vi "S2C_CheckBuildScript.vi"(8 "Error In":errorcluster, 11 "Entry":string) -> (0 "Error Out":errorcluster, 3 "Data":string[](array[string]))   [LabVIEW 2015]
doc: "Converts a script line entry into an executable table entry."
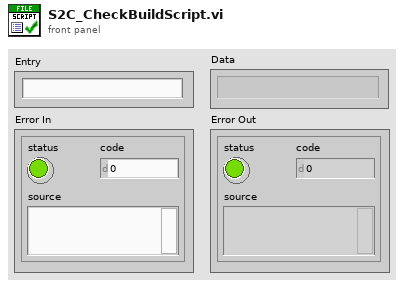
[diagram p1: front panel]
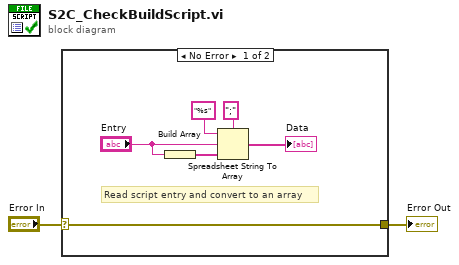
[diagram p0: block diagram]
diagram:
  n1 = case shown="No Error" "Error In" {
    selector: "Error In" -> [w4 w9]
    tunnel: [w4 w9] -> w1
    frame No Error {
      # "Read script entry and convert to an array"
      n2 = Build Array("Entry") -> (w6:string[])
      n3 = Spreadsheet String To Array(delimiter (Tab)=";", format string="%s", spreadsheet string="Entry", array type (2D Dbl)=w6) -> (array=→"Data":string[])
    }
    frame Error {
    }
  }
  "Error Out" <- w1
